vi "WTIME.vi"(10 "Incoming Data in":u8[](array[numeric])) -> (1 "CONFIG":u8, 2 "WTIME":u8)   [LabVIEW 2016, in "AMS TS3472 Light Sensor.lvlib" / "AMS TCS3472.lvclass"]
uses:
  AMS TCS3472.lvclass
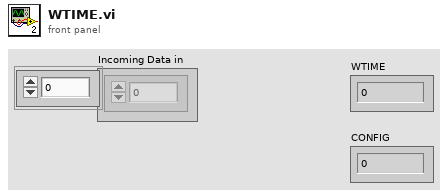
[diagram p1: front panel]
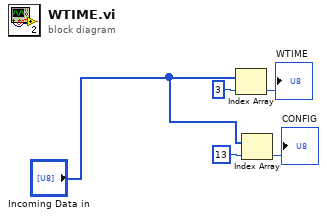
[diagram p0: block diagram]
diagram:
  n1 = Index Array(array="Incoming Data in", index=3) -> (element=→"WTIME":u8)
  n2 = Index Array(array="Incoming Data in", index=13) -> (element=→"CONFIG":u8)
